vi "DQMH Set Runtime Menu.vi"(7 "Module Disk Path":path, 8 "error in (no error)":errorcluster, 10 "Path to .rtm file":path, 11 "Application reference":refnum<vi>) -> (0 "error out":errorcluster)   [LabVIEW 2020, in "hse-dqmh-dynamicrequesters.lvlib"]
doc: "Calls the \"Set Runtime Menu\" request VI of the module in <b>Path to module directory</b>. Hands over the <b>Path to .rtm file</b>.\n\n____\nHAMPEL SOFTWARE ENGINEERING v3.8.0 (2023-12-18 14:41)"
uses:
  hse-dqmh-dynamicrequesters.lvlib
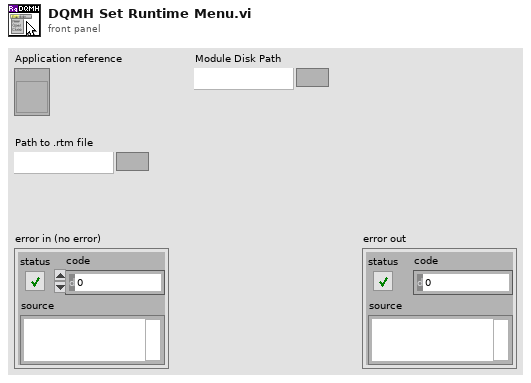
[diagram p1: front panel]
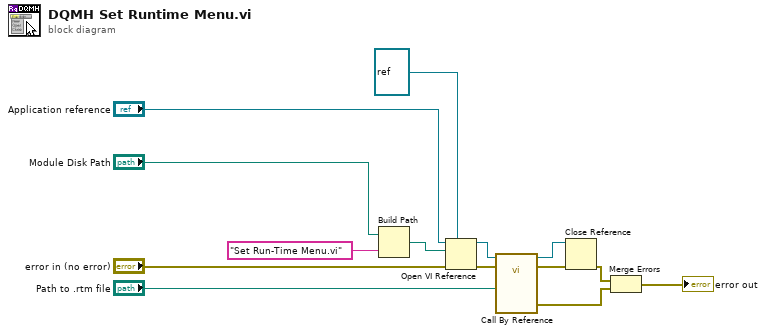
[diagram p0: block diagram]
diagram:
  n1 = Build Path(base path="Module Disk Path", name or relative path="Set Run-Time Menu.vi") -> (appended path=w10:path)
  n2 = Open VI Reference(type specifier VI Refnum (for type only)=refnum<vi> refnum, application reference (local)="Application reference", vi path=w10, error in (no error)="error in (no error)") -> (vi reference=w13:refnum<vi>, error out=w8:errorcluster)  [unwired: 2 in]
  n3 = call-by-ref "?"(reference=w13, error in=w8, "Run-Time Menu Path"="Path to .rtm file") -> (reference out=w2:refnum<vi>, error out=w4:errorcluster, 0:"error out"=w9:errorcluster)  [unwired: 10 in]
  n4 = Close Reference(reference=w2, error in (no error)=w4) -> (error out=w3:errorcluster)
  n5 = Merge Errors(w3, w9) -> (→"error out":errorcluster)
